vi "20180515mic_testing.vi"(9 "limit2":path=path "F:/ATE音频测试最终程序/20170720判断mic/limit2.txt" caption="上/下限路径", 10 "limit0":path=path "F:/ATE音频测试最终程序/20170720判断mic/limit0.txt" caption="上/下限路径", 11 "音源文件夹路径":path=path "C:/Users/Lenovo/Desktop/c12板子3210版本测试mic和spk/mic12均正负极接反/fangmic1") -> (0 "重测":bool, 1 "pass":bool=TRUE)   [LabVIEW 2014]
uses:
  <vilib>/drjdpowell/SQLite Library/SQL Statement/SQL Statement.lvclass/SQL Statement.ctl
  <vilib>/drjdpowell/SQLite Library/SQL Connection/Open (path).vi
  <vilib>/Utility/file.llb/Read From Spreadsheet File (DBL).vi
  <vilib>/Waveform/WDTOps.llb/WDT Index Channel DBL.vi
  <vilib>/measure/maspectr.llb/FFT Spectrum (Mag-Phase) for 1 Chan.vi
  <vilib>/measure/mamon.llb/Create Continuous Mask.vi
  <vilib>/measure/mamon.llb/Limit Testing Frequency.vi
  <vilib>/measure/maspectr.llb/FFT Spectrum (Real-Im) for 1 Chan.vi
  <vilib>/AdvancedString/Path To Command Line String.vi
  <vilib>/drjdpowell/SQLite Library/SQL Connection/Open (string).vi
  <vilib>/drjdpowell/SQLite Library/SQL Connection/Connection.lvclass
  <vilib>/measure/NI_MAPro.lvlib
  <vilib>/drjdpowell/SQLite Library/SQL Statement/SQL Statement.lvclass
panel:
  out "数组":dbl[](array[numeric])=[-21.861504748666253, -39.55147185823657, -75.68301687500698, -20.373611457828325]
  in  "路径":path=path "D:/pass/ate.wav"
  in  "error in (no error)":errorcluster
  out "error out":errorcluster
  out "ConnectionString 2":string="INSERT INTO ate(程序版本信息,测试时间,判定结果,计算值)   values('20180515_GVC3210MIC测试','2018年5月15日14-40-57','总fail,4pass,1fail,2fail,3pass,mic未接入或正负极接反或错位','-22,-40,-76,-20,');"
  out "单向mic 合格显示  2":bool[](array[boolean])
  out "音源文件名 1":string[](array[string])=["micrec1.wav"]
  in  "limit1":path=path "F:/ATE音频测试最终程序/20170720判断mic/limit1.txt" caption="上/下限路径"
  in  "分隔符 (\\t) 2":string=" " caption="分隔符(\\t)"
  in  "重测":bool
  in  "停止":bool
  out "错位":bool
  out "字符串":string="请检查是否存在mic未接入/正负极接反/错位等情况！"
  in  "分隔符 (\\t)":string=" " caption="分隔符(\\t)"
  out "J1203":bool
  out "J1202":bool
  out "J1201":bool
  out "J1204":bool
  out "单向mic 合格显示":bool[](array[boolean])=[TRUE]
  out "全向mic 合格显示":bool[](array[boolean])=[FALSE, TRUE]
  out "音源文件名 0":string[](array[string])=["micrec0.wav"]
  out "音源文件名2/3":string[](array[string])=["micrec2.wav", "micrec3.wav"]
  # "音频分析"
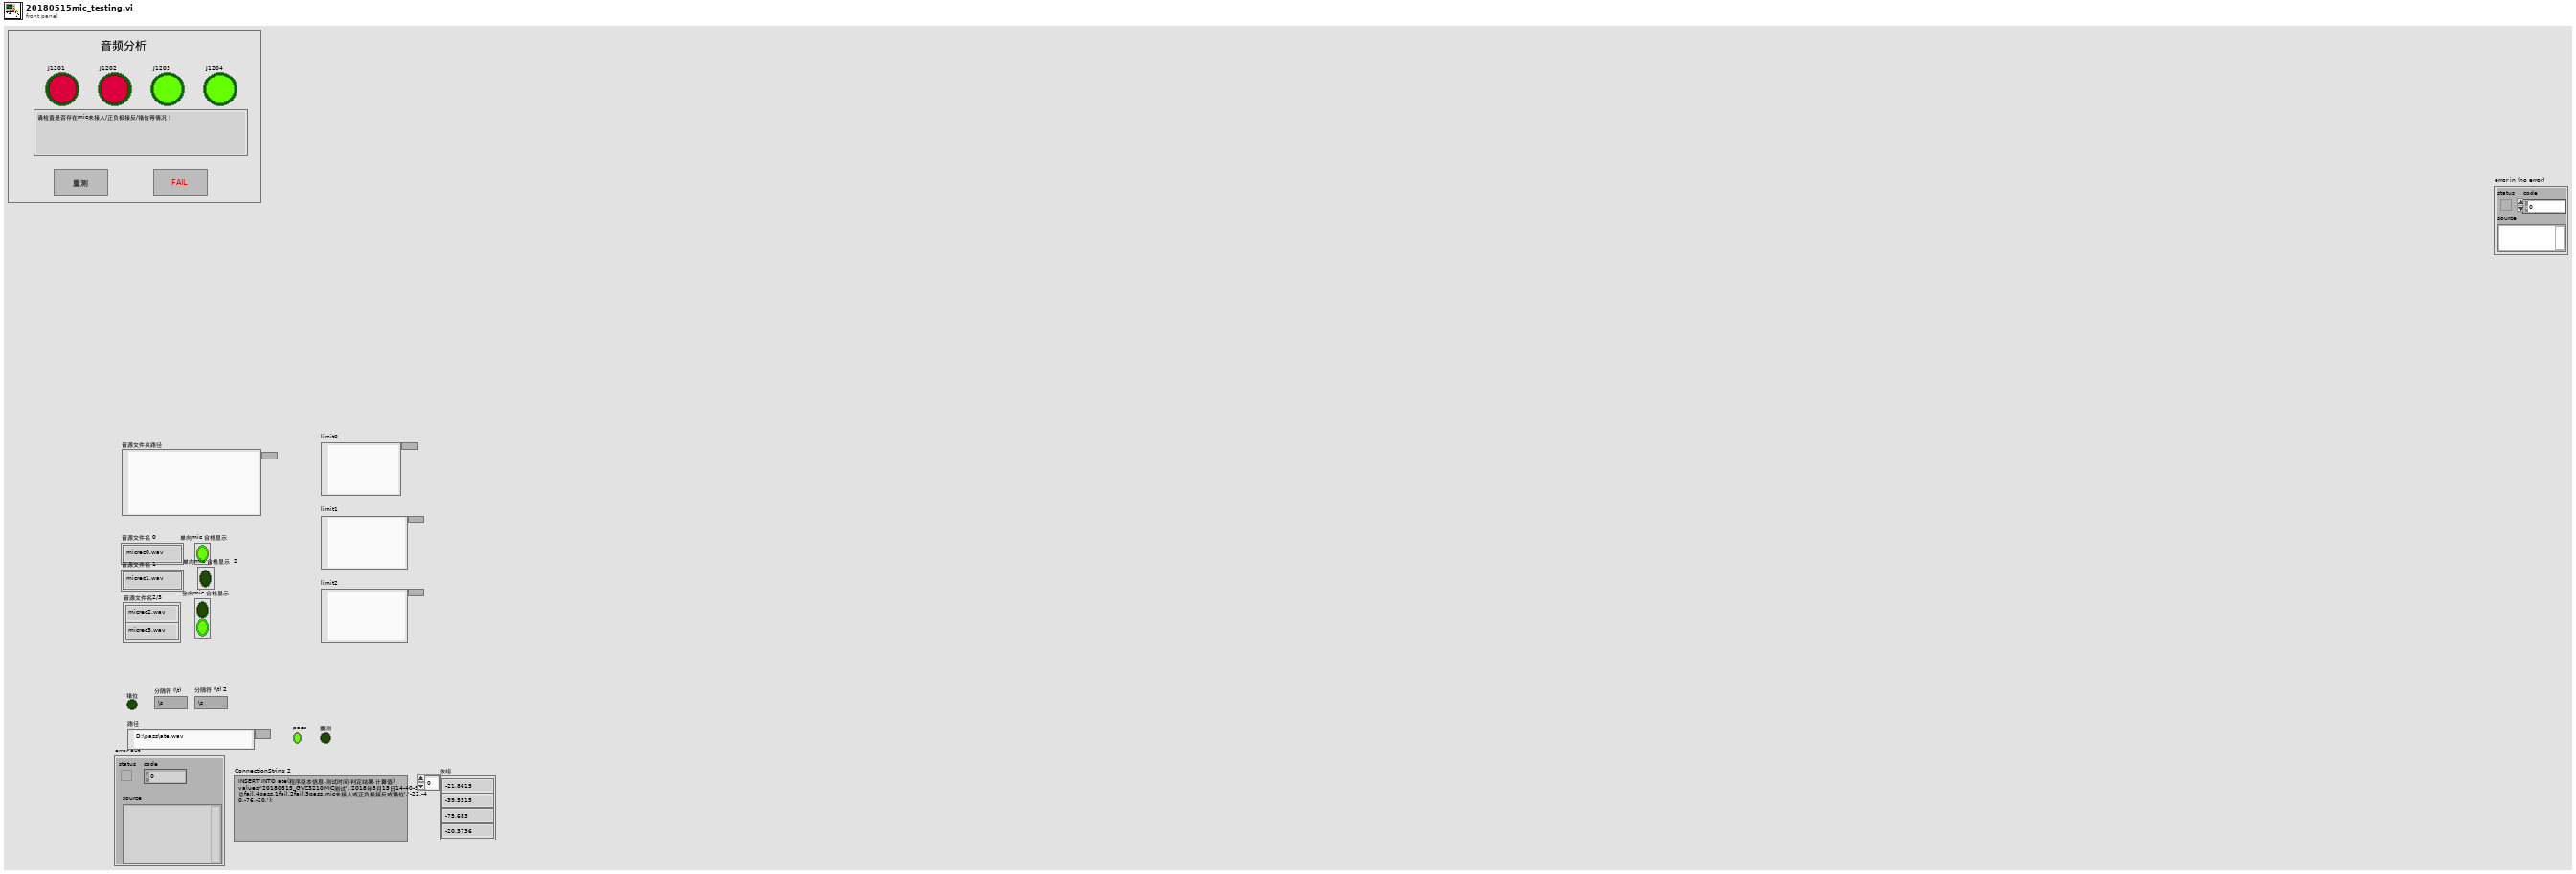
[diagram p1: front panel]
types:
  T1 = cluster{"averaging mode":enum16{"No averaging", "Vector averaging", "RMS averaging", "Peak hold"}, "weighting mode":enum16{"Linear", "Exponential"}, "number of averages":u32}
  T2 = cluster{"dB On (F)":bool, "unwrap phase (F)":bool, "convert to degree (F)":bool}
  T3 = cluster{"f0":dbl, "df":dbl, "imaginary part":dbl[]}
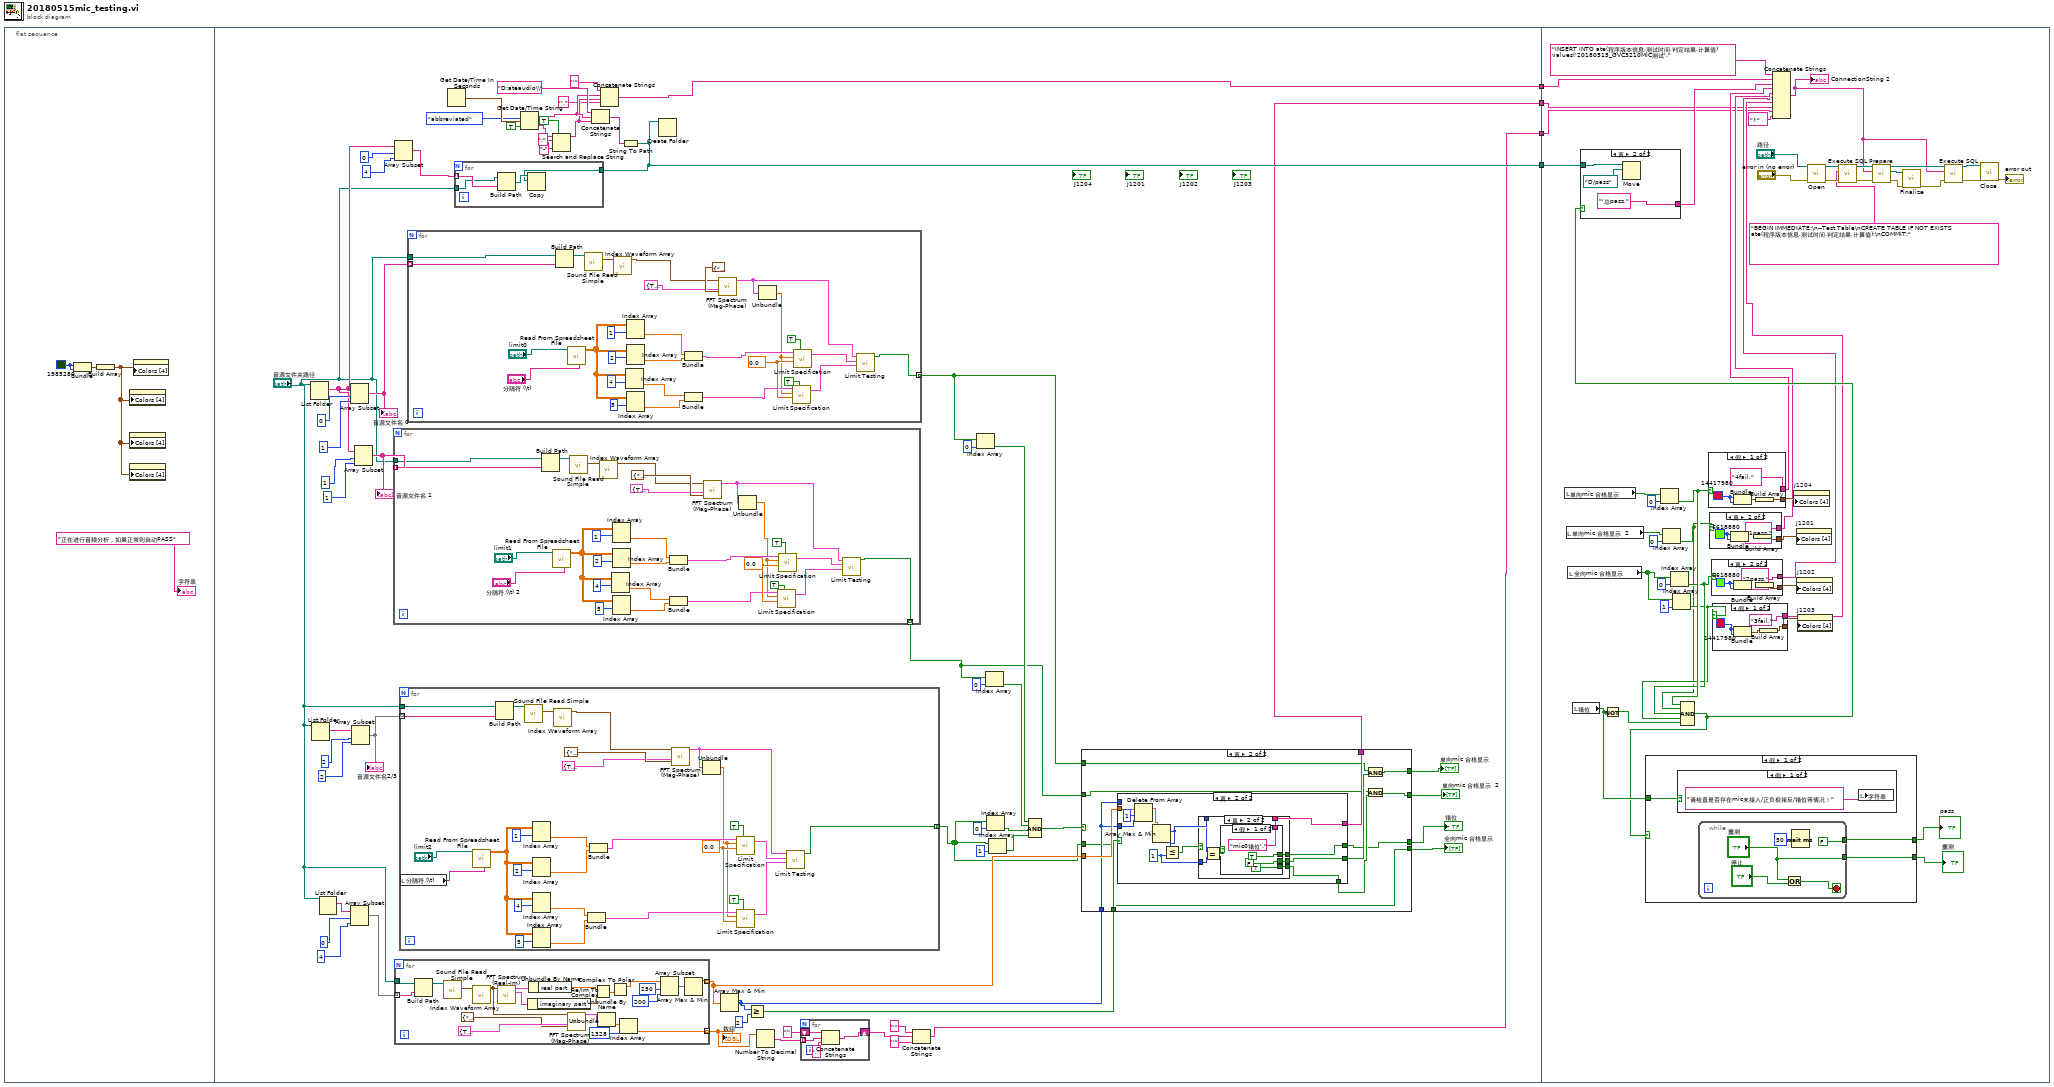
[diagram p0: block diagram]
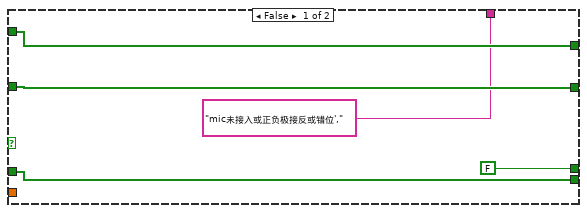
[diagram p2: hidden frame]
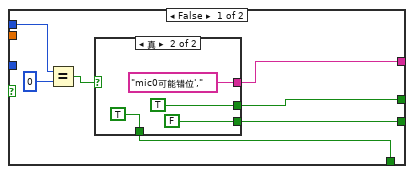
[diagram p3: hidden frame]
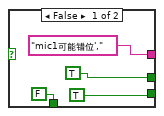
[diagram p4: hidden frame]
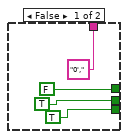
[diagram p5: hidden frame]
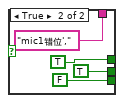
[diagram p6: hidden frame]
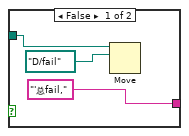
[diagram p7: hidden frame]
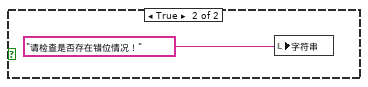
[diagram p8: hidden frame]
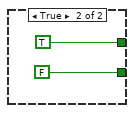
[diagram p9: hidden frame]
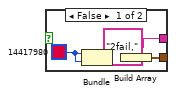
[diagram p10: hidden frame]
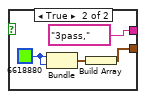
[diagram p11: hidden frame]
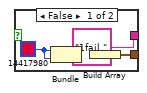
[diagram p12: hidden frame]
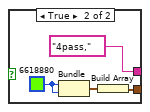
[diagram p13: hidden frame]
diagram:
  n1 = flat-sequence {
    tunnel: [w48] -> w4
    tunnel: [w43] -> w3
    tunnel: [w24] -> w2
    tunnel: [w9] -> w1
    tunnel: w4 -> [w269]
    tunnel: w3 -> [w270]
    tunnel: w2 -> [w248]
    tunnel: w1 -> [w246]
    frame #0 {
      w7 = u32 1985280 ("Color Box")
      n2 = Bundle("Color Box"=w7, "Color Box"=w7) -> (w8:cluster{"Color Box":u32, "Color Box":u32})  [unwired: 1 out]
      n3 = Build Array(w8) -> (w6:cluster{"Color Box":u32, "Color Box":u32}[])
      n4 = property on="J1202" class="Bool (严格)"("Colors [4]"=w6) -> ()  [unwired: 2 in, 2 out]
      n5 = property on="J1201" class="Bool (严格)"("Colors [4]"=w6) -> ()  [unwired: 2 in, 2 out]
      n6 = property on="J1204" class="Bool (严格)"("Colors [4]"=w6) -> ()  [unwired: 2 in, 2 out]
      n7 = property on="J1203" class="Bool (严格)"("Colors [4]"=w6) -> ()  [unwired: 2 in, 2 out]
      "字符串" <- "正在进行音频分析，如果正常则自动PASS" ("字符串")
    }
    frame #1 {
      n8 = List Folder(path="音源文件夹路径") -> (filenames=w49:string[])  [unwired: 1 in, 5 out]
      n9 = List Folder(path="音源文件夹路径") -> (filenames=w67:string[])  [unwired: 1 in, 5 out]
      n10 = List Folder(path="音源文件夹路径") -> (filenames=w42:string[])  [unwired: 1 in, 5 out]
      n11 = Array Subset(array=w49, index=0 ("索引"), length=1 ("长度")) -> (w68:string[])
      "音源文件名 0" <- w68
      n12 = Array Subset(array=w42, index=0 ("索引"), length=4 ("长度")) -> (w39:string[])
      n13 = Array Subset(array=w67, index=2 ("索引"), length=2 ("长度")) -> (w64:string[])
      "音源文件名2/3" <- w64
      n14 = Array Subset(array=w49, index=1 ("索引"), length=1 ("长度")) -> (w50:string[])
      "音源文件名 1" <- w50
      n15 = for {
        tunnel: "音源文件夹路径" -> [w162]
        tunnel: w50 -> [w164] mode=indexing
        tunnel: [w158] -> w20 mode=indexing
        w185 = 0.0 ("x0")
        n16 = Build Path(base path=w162, name or relative path=w164) -> (appended path=w163:path)
        n17 = call-poly <vilib>:"Read From Spreadsheet File.vi"("delimiter (\\t)"="分隔符 (\\t) 2", "file path (dialog if empty)"="limit1") -> ("all rows"=w167:dbl[][])  [unwired: 3 in, 6 out]
        n18 = call <vilib>:"Sound File Read Simple.vi"("path"=w163) -> ("data"=w182:waveform(dbl)[])  [unwired: 4 in, 6 out]
        n19 = call-poly <vilib>:"Index Waveform Array.vi"("waveform array"=w182) -> ("waveform"=w159:waveform(dbl))  [unwired: 2 in, 8 out]
        n20 = Index Array(array=w167, index (row)=4 ("索引 (行)")) -> (element=w169:dbl[])  [unwired: 1 in]
        n21 = Index Array(array=w167, index (row)=1 ("索引 (行)")) -> (element=w171:dbl[])  [unwired: 1 in]
        n22 = Index Array(array=w167, index (row)=2 ("索引 (行)")) -> (element=w170:dbl[])  [unwired: 1 in]
        n23 = Index Array(array=w167, index (row)=5 ("索引 (行)")) -> (element=w168:dbl[])  [unwired: 1 in]
        n24 = Bundle("all rows"=w171, "all rows"=w170) -> (w165:cluster{"all rows":dbl[], "all rows":dbl[]})  [unwired: 1 out]
        n25 = Bundle("all rows"=w169, "all rows"=w168) -> (w166:cluster{"all rows":dbl[], "all rows":dbl[]})  [unwired: 1 out]
        n26 = call-poly <vilib>:"FFT Spectrum (Mag-Phase).vi"("averaging parameters"=T1 {"averaging mode"=enum."No averaging", "weighting mode"=enum."Exponential", "number of averages"=10}, "view"=T2 {"dB On (F)"=TRUE, "unwrap phase (F)"=TRUE, "convert to degree (F)"=TRUE}, "time signal"=w159) -> ("magnitude"=w161:cluster{"f0":dbl, "df":dbl, "magnitude":dbl[]})  [unwired: 4 in, 4 out]
        n27 = Unbundle(w161) -> ("df"=w160:dbl)  [unwired: 2 out]
        n28 = call-poly <vilib>:"Limit Specification.vi"("Specification Cluster"=w166, "dx"=w160, "x0"=w185, "Reset"=TRUE) -> ("Limit"=w178:cluster{"x0":dbl, "dx":dbl, "Y":dbl[]})  [unwired: 1 in, 1 out]
        n29 = call-poly <vilib>:"Limit Specification.vi"("Specification Cluster"=w165, "dx"=w160, "x0"=w185, "Reset"=TRUE) -> ("Limit"=w179:cluster{"x0":dbl, "dx":dbl, "Y":dbl[]})  [unwired: 1 in, 1 out]
        n30 = call-poly <vilib>:"Limit Testing.vi"("lower limit"=w178, "upper limit"=w179, "signal in"=w161) -> ("test passed?"=w158:bool)  [unwired: 2 in, 6 out]
      }
      n31 = Array Subset(array=w49, index=0 ("索引"), length=4 ("长度")) -> (w53:string[])
      n32 = for {
        tunnel: w39 -> [w155] mode=indexing
        tunnel: [w147] -> w26 mode=indexing
        tunnel: "音源文件夹路径" -> [w144]
        tunnel: [w137] -> w15 mode=indexing
        n33 = Build Path(base path=w144, name or relative path=w155) -> (appended path=w156:path)
        n34 = call <vilib>:"Sound File Read Simple.vi"("path"=w156) -> ("data"=w157:waveform(dbl)[])  [unwired: 4 in, 6 out]
        n35 = call-poly <vilib>:"Index Waveform Array.vi"("waveform array"=w157) -> ("waveform"=w140:waveform(dbl))  [unwired: 2 in, 8 out]
        n36 = call-poly <vilib>:"FFT Spectrum (Real-Im).vi"("time signal"=w140) -> ("imaginary part"=w151:T3, "real part"=w145:cluster{"f0":dbl, "df":dbl, "real part":dbl[]})  [unwired: 5 in, 4 out]
        n37 = Unbundle By Name(w151) -> ("imaginary part"=w153:dbl[])
        n38 = Unbundle By Name(w145) -> ("real part"=w152:dbl[])
        n39 = call-poly <vilib>:"FFT Spectrum (Mag-Phase).vi"("averaging parameters"=T1 {"averaging mode"=enum."No averaging", "weighting mode"=enum."Exponential", "number of averages"=10}, "view"=T2 {"dB On (F)"=TRUE, "unwrap phase (F)"=TRUE, "convert to degree (F)"=TRUE}, "time signal"=w140) -> ("magnitude"=w143:cluster{"f0":dbl, "df":dbl, "magnitude":dbl[]})  [unwired: 4 in, 4 out]
        n40 = Re/Im To Complex(1:w153, 2:w152) -> (0:w154:cdb[])
        n41 = Unbundle(w143) -> ("magnitude"=w139:dbl[])  [unwired: 2 out]
        n42 = Complex To Polar(r * e^(i*theta)=w154) -> (r=w146:dbl[])  [unwired: 1 out]
        n43 = Index Array(array=w139, index=1328 ("索引")) -> (element=w137:dbl)
        n44 = Array Subset(array=w146, index=250 ("索引"), length=200 ("长度")) -> (w150:dbl[])
        n45 = Array Max & Min(array=w150) -> (max value=w147:dbl)  [unwired: 3 out]
      }
      "数组" <- w15
      n46 = for {
        tunnel: w64 -> [w207] mode=indexing
        tunnel: "音源文件夹路径" -> [w213]
        tunnel: [w190] -> w18 mode=indexing
        w217 = 0.0 ("x0")
        n47 = local read "分隔符 (\\t)"() -> (w193:string)
        n48 = call-poly <vilib>:"Read From Spreadsheet File.vi"("delimiter (\\t)"=w193, "file path (dialog if empty)"="limit2") -> ("all rows"=w196:dbl[][])  [unwired: 3 in, 6 out]
        n49 = Build Path(base path=w213, name or relative path=w207) -> (appended path=w214:path)
        n50 = call <vilib>:"Sound File Read Simple.vi"("path"=w214) -> ("data"=w212:waveform(dbl)[])  [unwired: 4 in, 6 out]
        n51 = Index Array(array=w196, index (row)=1 ("索引 (行)")) -> (element=w200:dbl[])  [unwired: 1 in]
        n52 = Index Array(array=w196, index (row)=2 ("索引 (行)")) -> (element=w199:dbl[])  [unwired: 1 in]
        n53 = Index Array(array=w196, index (row)=4 ("索引 (行)")) -> (element=w198:dbl[])  [unwired: 1 in]
        n54 = Index Array(array=w196, index (row)=5 ("索引 (行)")) -> (element=w197:dbl[])  [unwired: 1 in]
        n55 = call-poly <vilib>:"Index Waveform Array.vi"("waveform array"=w212) -> ("waveform"=w206:waveform(dbl))  [unwired: 2 in, 8 out]
        n56 = Bundle("all rows"=w198, "all rows"=w197) -> (w194:cluster{"all rows":dbl[], "all rows":dbl[]})  [unwired: 1 out]
        n57 = Bundle("all rows"=w200, "all rows"=w199) -> (w195:cluster{"all rows":dbl[], "all rows":dbl[]})  [unwired: 1 out]
        n58 = call-poly <vilib>:"FFT Spectrum (Mag-Phase).vi"("averaging parameters"=T1 {"averaging mode"=enum."No averaging", "weighting mode"=enum."Exponential", "number of averages"=10}, "view"=T2 {"dB On (F)"=TRUE, "unwrap phase (F)"=TRUE, "convert to degree (F)"=TRUE}, "time signal"=w206) -> ("magnitude"=w192:cluster{"f0":dbl, "df":dbl, "magnitude":dbl[]})  [unwired: 4 in, 4 out]
        n59 = Unbundle(w192) -> ("df"=w191:dbl)  [unwired: 2 out]
        n60 = call-poly <vilib>:"Limit Specification.vi"("Specification Cluster"=w195, "dx"=w191, "x0"=w217, "Reset"=TRUE) -> ("Limit"=w209:cluster{"x0":dbl, "dx":dbl, "Y":dbl[]})  [unwired: 1 in, 1 out]
        n61 = call-poly <vilib>:"Limit Specification.vi"("Specification Cluster"=w194, "dx"=w191, "x0"=w217, "Reset"=TRUE) -> ("Limit"=w208:cluster{"x0":dbl, "dx":dbl, "Y":dbl[]})  [unwired: 1 in, 1 out]
        n62 = call-poly <vilib>:"Limit Testing.vi"("lower limit"=w208, "upper limit"=w209, "signal in"=w192) -> ("test passed?"=w190:bool)  [unwired: 2 in, 6 out]
      }
      n63 = for {
        tunnel: "音源文件夹路径" -> [w223]
        tunnel: w68 -> [w225] mode=indexing
        tunnel: [w218] -> w21 mode=indexing
        w245 = 0.0 ("x0")
        n64 = Build Path(base path=w223, name or relative path=w225) -> (appended path=w224:path)
        n65 = call-poly <vilib>:"Read From Spreadsheet File.vi"("delimiter (\\t)"="分隔符 (\\t)", "file path (dialog if empty)"="limit0") -> ("all rows"=w227:dbl[][])  [unwired: 3 in, 6 out]
        n66 = call <vilib>:"Sound File Read Simple.vi"("path"=w224) -> ("data"=w242:waveform(dbl)[])  [unwired: 4 in, 6 out]
        n67 = call-poly <vilib>:"Index Waveform Array.vi"("waveform array"=w242) -> ("waveform"=w219:waveform(dbl))  [unwired: 2 in, 8 out]
        n68 = Index Array(array=w227, index (row)=4 ("索引 (行)")) -> (element=w229:dbl[])  [unwired: 1 in]
        n69 = Index Array(array=w227, index (row)=1 ("索引 (行)")) -> (element=w231:dbl[])  [unwired: 1 in]
        n70 = Index Array(array=w227, index (row)=2 ("索引 (行)")) -> (element=w230:dbl[])  [unwired: 1 in]
        n71 = Index Array(array=w227, index (row)=5 ("索引 (行)")) -> (element=w228:dbl[])  [unwired: 1 in]
        n72 = Bundle("all rows"=w231, "all rows"=w230) -> (w226:cluster{"all rows":dbl[], "all rows":dbl[]})  [unwired: 1 out]
        n73 = Bundle("all rows"=w229, "all rows"=w228) -> (w222:cluster{"all rows":dbl[], "all rows":dbl[]})  [unwired: 1 out]
        n74 = call-poly <vilib>:"FFT Spectrum (Mag-Phase).vi"("averaging parameters"=T1 {"averaging mode"=enum."No averaging", "weighting mode"=enum."Exponential", "number of averages"=10}, "view"=T2 {"dB On (F)"=TRUE, "unwrap phase (F)"=TRUE, "convert to degree (F)"=TRUE}, "time signal"=w219) -> ("magnitude"=w221:cluster{"f0":dbl, "df":dbl, "magnitude":dbl[]})  [unwired: 4 in, 4 out]
        n75 = Unbundle(w221) -> ("df"=w220:dbl)  [unwired: 2 out]
        n76 = call-poly <vilib>:"Limit Specification.vi"("Specification Cluster"=w222, "dx"=w220, "x0"=w245, "Reset"=TRUE) -> ("Limit"=w238:cluster{"x0":dbl, "dx":dbl, "Y":dbl[]})  [unwired: 1 in, 1 out]
        n77 = call-poly <vilib>:"Limit Specification.vi"("Specification Cluster"=w226, "dx"=w220, "x0"=w245, "Reset"=TRUE) -> ("Limit"=w239:cluster{"x0":dbl, "dx":dbl, "Y":dbl[]})  [unwired: 1 in, 1 out]
        n78 = call-poly <vilib>:"Limit Testing.vi"("lower limit"=w238, "upper limit"=w239, "signal in"=w221) -> ("test passed?"=w218:bool)  [unwired: 2 in, 6 out]
      }
      n79 = Get Date/Time In Seconds() -> (seconds since 1Jan1904=w60:timestamp)
      n80 = Get Date/Time String(date format (0)=enum16{"short", "long", "abbreviated"}."abbreviated" ("日期格式(0)"), seconds (now)=w60, want seconds? (F)=TRUE ("需要秒？(F)")) -> (date string=w47:string, time string=w57:string)
      n81 = Search and Replace String(replace all?=TRUE ("替换全部？(F)"), input string=w57, search string=":" ("搜索字符串"), replace string="-" ("替换字符串(\"\")")) -> (result string=w46:string)  [unwired: 1 in, 6 out]
      n82 = Concatenate Strings("D:ateaudio\\" ("字符串"), w47, w46) -> (w29:string)
      n83 = Concatenate Strings("'" ("替换字符串(\"\")"), w47, w46, "'," ("替换字符串(\"\")")) -> (w43:string)
      n84 = String To Path(string=w29) -> (path=w48:path)
      n85 = for {
        tunnel: w53 -> [w189] mode=indexing
        tunnel: "音源文件夹路径" -> [w188]
        tunnel: w48 -> [w186]
        n86 = Build Path(base path=w188, name or relative path=w189) -> (appended path=w187:path)
        n87 = Copy(10:w186, 11:w187) -> ()  [unwired: 1 in, 5 out]
      }
      n88 = Create Folder(path (use dialog)=w48) -> ()  [unwired: 1 in, 4 out]
      n89 = Array Max & Min(array=w26) -> (max index (indices)=w25:i32)  [unwired: 3 out]
      n90 = Greater Or Equal?(x=w25, y=2) -> (x >= y?=w27:bool)
      n91 = Number To Decimal String(number=w15) -> (decimal integer string=w14:string[])  [unwired: 1 in]
      n92 = for {
        tunnel: w14 -> [w72] mode=indexing
        shift-right: [w73] -> w12
        shift-left: "" -> [w74]
        n93 = Concatenate Strings(w74, w72, ",") -> (w73:string)
      }
      n94 = Concatenate Strings("'", w12, "'") -> (w9:string)
      n95 = Index Array(array=w21, index=0 ("索引")) -> (element=w23:bool)
      n96 = Index Array(array=w20, index=0 ("索引")) -> (element=w30:bool)
      n97 = Index Array(array=w18, index=0 ("索引")) -> (element=w34:bool)
      n98 = Index Array(array=w18, index=1 ("索引")) -> (element=w33:bool)
      n99 = Compound Arithmetic op=AND(w23, w30, w34, w33) -> (w28:bool)
      n100 = case shown="真" w28 {
        tunnel: w27 -> [_ w91]
        tunnel: w26 -> [_ w90]
        tunnel: w25 -> [_ w89]
        tunnel: ["mic未接入或正负极接反或错位'," w88] -> w24
        tunnel: w21 -> [w79 w87]
        tunnel: [w79 w85] -> w22
        tunnel: w20 -> [w78 w84]
        tunnel: [w78 w82] -> w19
        tunnel: w18 -> [w77 w81]
        tunnel: [w77 w81] -> w17
        tunnel: [FALSE w80] -> w16
        frame False {
        }
        frame True {
          n101 = case shown="真" w91 {
            tunnel: [w95 w110] -> w80
            tunnel: [w96 w107] -> w88
            tunnel: [w94 w108] -> w86
            tunnel: [w93 w109] -> w83
            tunnel: w90 -> [_ w117]
            tunnel: w89 -> [_ w115]
            tunnel: w89 -> [w92 _]
            frame False {
              n102 = Equal?(x=w92, y=0) -> (x = y?=w97:bool)
              n103 = case shown="真" w97 {
                tunnel: ["mic1可能错位'," "mic0可能错位',"] -> w96
                tunnel: [TRUE ("Reset") TRUE ("Reset")] -> w95
                tunnel: [TRUE ("Reset") FALSE ("Reset")] -> w94
                tunnel: [FALSE ("Reset") TRUE ("Reset")] -> w93
                frame False {
                }
                frame True {
                }
              }
            }
            frame True {
              w111 = 1 ("y")
              n104 = Delete From Array(array=w117, length=1 ("长度"), index=w115) -> (array with subset deleted=w114:dbl[])  [unwired: 1 out]
              n105 = Array Max & Min(array=w114) -> (max index (indices)=w112:i32)  [unwired: 3 out]
              n106 = Less Or Equal?(x=w112, y=w111) -> (x <= y?=w113:bool)
              n107 = case shown="真" w113 {
                tunnel: w112 -> [_ w128]
                tunnel: w111 -> [_ w127]
                tunnel: [FALSE w125] -> w110
                tunnel: [TRUE w124] -> w109
                tunnel: [TRUE w123] -> w108
                tunnel: ["0'," w122] -> w107
                frame False {
                }
                frame True {
                  n108 = Equal?(x=w128, y=w127) -> (x = y?=w126:bool)
                  n109 = case shown="假" w126 {
                    tunnel: [TRUE ("Reset") TRUE] -> w125
                    tunnel: [TRUE ("Reset") FALSE ("Reset")] -> w124
                    tunnel: [FALSE ("Reset") TRUE ("Reset")] -> w123
                    tunnel: ["mic0错位'," "mic1错位',"] -> w122
                    frame False {
                    }
                    frame True {
                    }
                  }
                }
              }
            }
          }
          n110 = And(x=w87, y=w86) -> (x .and. y?=w85:bool[])
          n111 = And(x=w84, y=w83) -> (x .and. y?=w82:bool[])
        }
      }
      "全向mic 合格显示" <- w17
      "单向mic 合格显示" <- w22
      "单向mic 合格显示  2" <- w19
      "错位" <- w16
    }
    frame #2 {
      n112 = local read "单向mic 合格显示"() -> (w290:bool[])
      n113 = local read "单向mic 合格显示  2"() -> (w274:bool[])
      n114 = local read "全向mic 合格显示"() -> (w287:bool[])
      n115 = local read "错位"() -> (w278:bool)
      n116 = Not(x=w278) -> (.not. x?=w279:bool)
      n117 = Index Array(array=w290, index=0 ("索引")) -> (element=w282:bool)
      n118 = Index Array(array=w274, index=0 ("索引")) -> (element=w273:bool)
      n119 = Index Array(array=w287, index=0 ("索引")) -> (element=w281:bool)
      n120 = Index Array(array=w287, index=1 ("索引")) -> (element=w280:bool)
      n121 = Compound Arithmetic op=AND(w282, w273, w281, w280, w279) -> (w272:bool)
      n122 = case shown="真" w272 {
        tunnel: w269 -> [w293 w297]
        tunnel: ["'总fail," "'总pass,"] -> w249
        frame False {
          n123 = Move(source path=w293, 10:path "D:/fail" ("目标路径（使用对话框）")) -> ()  [unwired: 3 in, 3 out]
        }
        frame True {
          n124 = Move(source path=w297, 10:path "D:/pass" ("目标路径（使用对话框）")) -> ()  [unwired: 3 in, 3 out]
        }
      }
      n125 = case shown="假" w272 {
        tunnel: w278 -> [w300 _]
        tunnel: [w298 FALSE] -> w276
        tunnel: [w299 TRUE] -> w277
        frame False {
          n126 = case shown="假" w300 {
            frame False {
              n127 = local write "字符串"("请检查是否存在mic未接入/正负极接反/错位等情况！") -> ()
            }
            frame True {
              n128 = local write "字符串"("请检查是否存在错位情况！") -> ()
            }
          }
          n129 = while {
            tunnel: [FALSE] -> w299
            tunnel: ["重测"] -> w298
            stop <- w304 stop-if-true
            n130 = Or(x="重测", y="停止") -> (x .or. y?=w304:bool)
            n131 = Wait (ms)(milliseconds to wait=u32 50 ("等待时间（毫秒）")) -> ()  [unwired: 1 out]
          }
        }
        frame True {
        }
      }
      "pass" <- w277
      "重测" <- w276
      n132 = case shown="假" w282 {
        tunnel: [w336 w339] -> w286
        tunnel: ["4fail," "4pass,"] -> w268
        frame False {
          w335 = u32 14417980 ("Color Box")
          n133 = Bundle("Color Box"=w335, "Color Box"=w335) -> (w337:cluster{"Color Box":u32, "Color Box":u32})  [unwired: 1 out]
          n134 = Build Array(w337) -> (w336:cluster{"Color Box":u32, "Color Box":u32}[])
        }
        frame True {
          w340 = u32 6618880 ("Color Box")
          n135 = Bundle("Color Box"=w340, "Color Box"=w340) -> (w341:cluster{"Color Box":u32, "Color Box":u32})  [unwired: 1 out]
          n136 = Build Array(w341) -> (w339:cluster{"Color Box":u32, "Color Box":u32}[])
        }
      }
      n137 = case shown="真" w273 {
        tunnel: [w328 w331] -> w285
        tunnel: ["1fail," "1pass,"] -> w267
        frame False {
          w327 = u32 14417980 ("Color Box")
          n138 = Bundle("Color Box"=w327, "Color Box"=w327) -> (w329:cluster{"Color Box":u32, "Color Box":u32})  [unwired: 1 out]
          n139 = Build Array(w329) -> (w328:cluster{"Color Box":u32, "Color Box":u32}[])
        }
        frame True {
          w332 = u32 6618880 ("Color Box")
          n140 = Bundle("Color Box"=w332, "Color Box"=w332) -> (w333:cluster{"Color Box":u32, "Color Box":u32})  [unwired: 1 out]
          n141 = Build Array(w333) -> (w331:cluster{"Color Box":u32, "Color Box":u32}[])
        }
      }
      n142 = case shown="真" w281 {
        tunnel: [w312 w315] -> w284
        tunnel: ["2fail," "2pass,"] -> w266
        frame False {
          w311 = u32 14417980 ("Color Box")
          n143 = Bundle("Color Box"=w311, "Color Box"=w311) -> (w313:cluster{"Color Box":u32, "Color Box":u32})  [unwired: 1 out]
          n144 = Build Array(w313) -> (w312:cluster{"Color Box":u32, "Color Box":u32}[])
        }
        frame True {
          w316 = u32 6618880 ("Color Box")
          n145 = Bundle("Color Box"=w316, "Color Box"=w316) -> (w317:cluster{"Color Box":u32, "Color Box":u32})  [unwired: 1 out]
          n146 = Build Array(w317) -> (w315:cluster{"Color Box":u32, "Color Box":u32}[])
        }
      }
      n147 = case shown="假" w280 {
        tunnel: [w320 w323] -> w283
        tunnel: ["3fail," "3pass,"] -> w265
        frame False {
          w319 = u32 14417980 ("Color Box")
          n148 = Bundle("Color Box"=w319, "Color Box"=w319) -> (w321:cluster{"Color Box":u32, "Color Box":u32})  [unwired: 1 out]
          n149 = Build Array(w321) -> (w320:cluster{"Color Box":u32, "Color Box":u32}[])
        }
        frame True {
          w324 = u32 6618880 ("Color Box")
          n150 = Bundle("Color Box"=w324, "Color Box"=w324) -> (w325:cluster{"Color Box":u32, "Color Box":u32})  [unwired: 1 out]
          n151 = Build Array(w325) -> (w323:cluster{"Color Box":u32, "Color Box":u32}[])
        }
      }
      n152 = Concatenate Strings("INSERT INTO ate(程序版本信息,测试时间,判定结果,计算值)   values('20180515_GVC3210MIC测试'," ("字符串"), w270, w249, w268, w267, w266, w265, w248, w246, ");" ("字符串")) -> (w251:string)
      "ConnectionString 2" <- w251
      n153 = property on="J1204" class="Bool (严格)"("Colors [4]"=w286) -> ()  [unwired: 2 in, 2 out]
      n154 = property on="J1201" class="Bool (严格)"("Colors [4]"=w285) -> ()  [unwired: 2 in, 2 out]
      n155 = property on="J1202" class="Bool (严格)"("Colors [4]"=w284) -> ()  [unwired: 2 in, 2 out]
      n156 = property on="J1203" class="Bool (严格)"("Colors [4]"=w283) -> ()  [unwired: 2 in, 2 out]
      n157 = call-poly <vilib>:"Open.vi"("error in (no error)"="error in (no error)", "db file"="路径") -> ("error out"=w252:errorcluster, "SQLite Connection out"=w253:refnum<class "Connection.lvclass">)  [unwired: 8 in]
      n158 = call <vilib>:"Execute SQL.vi"("error in (no error)"=w252, "SQL"="BEGIN IMMEDIATE;\n--Test Table\nCREATE TABLE IF NOT EXISTS ate(程序版本信息,测试时间,判定结果,计算值);\nCOMMIT;", "SQLite Connection in"=w253) -> ("error out"=w254:errorcluster, "SQLite Connection out"=w257:refnum<class "Connection.lvclass">)  [unwired: 5 in, 2 out]
      n159 = call <vilib>:"Prepare.vi"("error in (no error)"=w254, "SQL"=w251, "SQLite Connection in"=w257) -> ("error out"=w263:errorcluster, "SQL Statement out"=w262:refnum<class "SQL Statement.lvclass">, "SQLite Connection out"=w261:refnum<class "Connection.lvclass">)  [unwired: 4 in, 2 out]
      n160 = call <vilib>:"Finalize.vi"("error in (no error)"=w263, "SQL Statement in"=w262) -> ("error out"=w264:errorcluster)  [unwired: 9 in]
      n161 = call <vilib>:"Execute SQL.vi"("error in (no error)"=w264, "SQL"=w251, "SQLite Connection in"=w261) -> ("error out"=w259:errorcluster, "SQLite Connection out"=w258:refnum<class "Connection.lvclass">)  [unwired: 5 in, 2 out]
      n162 = call <vilib>:"Close.vi"("error in (no error)"=w259, "SQLite Connection in"=w258) -> ("error out"=→"error out":errorcluster)  [unwired: 9 in]
    }
  }
